vi "StopCountdown.vi"(8 "error in":errorcluster, 11 "TimeoutID":u32) -> (0 "error out":errorcluster)   [LabVIEW 2020, in "Timer.lvlib"]
uses:
  Timer.lvlib
  TimeoutTask.vi
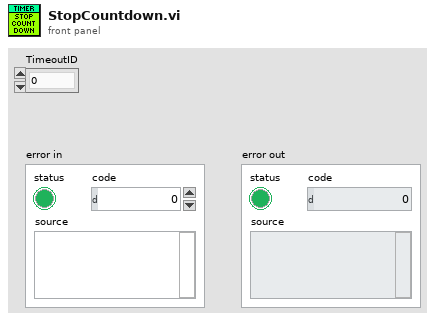
[diagram p1: front panel]
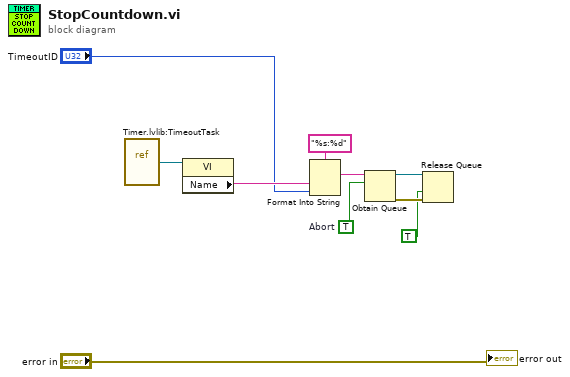
[diagram p0: block diagram]
diagram:
  w5 = TRUE  # Abort
  n1 = vi-ref "Timer.lvlib:TimeoutTask.vi"() -> (w8:refnum<vi>)
  n2 = property class="VI"(reference=w8) -> ("Name"=w4:string)  [unwired: 1 in, 2 out]
  n3 = Format Into String(format string="%s:%d", w4, "TimeoutID") -> (resulting string=w6:string)  [unwired: 2 in, 1 out]
  n4 = Obtain Queue(name (unnamed)=w6, element data type=w5) -> (queue out=w2:refnum<queue>, error out=w9:errorcluster)  [unwired: 3 in, 1 out]
  n5 = Release Queue(queue=w2, force destroy? (F)=TRUE, error in (no error)=w9) -> ()  [unwired: 3 out]
  "error out" <- "error in"
